vi "ChangeMainTap.vi"(2 "error in":errorcluster, 3 "ItemTag":string, 4 "reference":refnum<vi>) -> (0 "error out":errorcluster, 1 "Boolean":bool)   [LabVIEW 2013]
panel:
  out "Value":variant
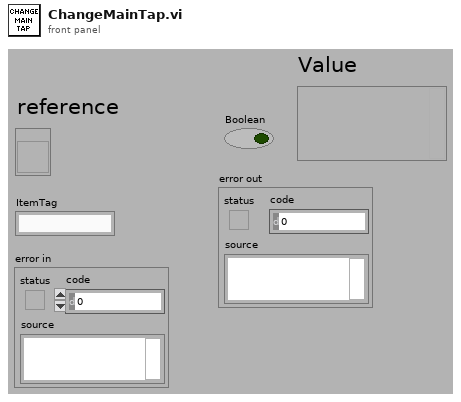
[diagram p1: front panel]
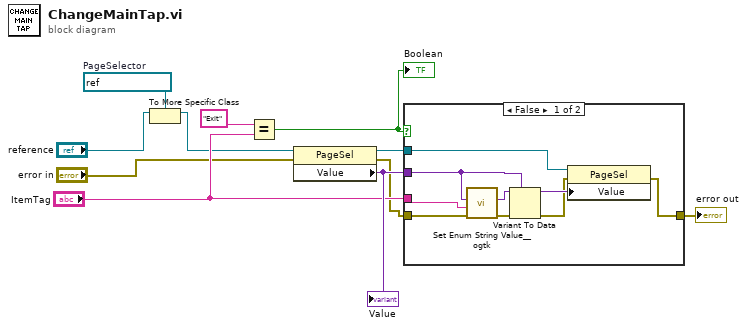
[diagram p0: block diagram]
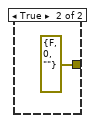
[diagram p2: hidden frame]
diagram:
  w4 = refnum<vi> refnum  # PageSelector
  n1 = To More Specific Class(target class=w4, reference="reference") -> (specific class reference=w3:refnum<vi>)  [unwired: 1 in, 1 out]
  n2 = Equal?(x="Exit", y="ItemTag") -> (x = y?=w7:bool)
  "Boolean" <- w7
  n3 = property class="PageSel"(reference=w3, error in="error in") -> (reference out=w11:refnum<vi>, error out=w1:errorcluster, "Value"=w10:variant)
  "Value" <- w10
  n4 = case shown="False" w7 {
    tunnel: w10 -> [w19 _]
    tunnel: "ItemTag" -> [w18 _]
    tunnel: [w12 errorcluster {"status"=FALSE, "code"=0, "source"=""} ("error out")] -> w8
    tunnel: w1 -> [w16 _]
    tunnel: w11 -> [w15 _]
    frame False {
      n5 = call <userlib>:"Set Enum String Value__ogtk.vi"("error in (no error)"=w16, "String Value"=w18, "Default Enum Value"=w19) -> ("error out"=w17:errorcluster, "Enum"=w20:variant)  [unwired: 7 in]
      n6 = Variant To Data(error in=w17, type=w19, Variant=w20) -> (data=w14:variant, error out=w13:errorcluster)
      n7 = property class="PageSel"(reference=w15, error in=w13, "Value"=w14) -> (error out=w12:errorcluster)  [unwired: 1 out]
    }
    frame True {
    }
  }
  "error out" <- w8
